vi "Trajectory Demo.vi"() -> ()   [LabVIEW 2017, in "NI_Kinematics.lvlib"]
uses:
  <vilib>/robotics/Kinematics/NI_Kinematics.lvlib
  <vilib>/robotics/Kinematics/Generate Joint Trajectory (Array).vi
  <vilib>/robotics/Kinematics/Robot/NI_Robotics_Serial Robot Arm.lvclass
panel:
  out "QDD":dbl[][](array[numeric])
  out "QD":dbl[][](array[numeric])
  out "Q":dbl[][](array[numeric])
  out "Time (ms)":u32
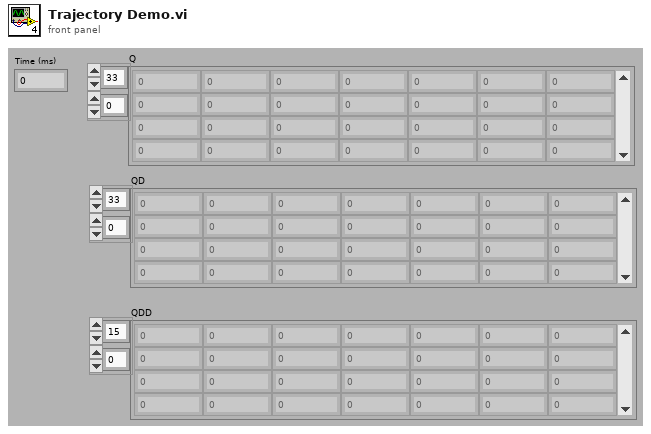
[diagram p1: front panel]
types:
  T1 = typedef "NI_Robotics_Serial Robot Arm.lvclass/Robot Pose.ctl" = cluster{"name":string, "description":string, "joint positions":dbl[]}
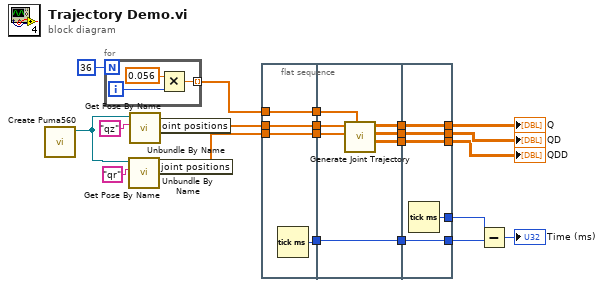
[diagram p0: block diagram]
diagram:
  n1 = call <vilib>:"Create Puma560.vi"() -> ("Puma560 Robot"=w21:refnum<class "NI_Robotics_Serial Robot Arm.lvclass">)  [unwired: 1 in, 10 out]
  n2 = for {
    N: 36 -> [_]
    tunnel: [w24] -> w12 mode=indexing
    i -> [w26]
    n3 = Multiply(x=0.056, y=w26) -> (x*y=w24:dbl)
  }
  n4 = call <vilib>:"Get Pose By Name.vi"("name"="qr" ("Name"), "serial arm in"=w21) -> ("serial arm pose"=w20:T1)  [unwired: 7 in, 2 out]
  n5 = call <vilib>:"Get Pose By Name.vi"("name"="qz" ("Name"), "serial arm in"=w21) -> ("serial arm pose"=w19:T1)  [unwired: 7 in, 2 out]
  n6 = Unbundle By Name(w19) -> ("joint positions"=w10:dbl[])
  n7 = Unbundle By Name(w20) -> ("joint positions"=w8:dbl[])
  n8 = flat-sequence {
    tunnel: [w30] -> w17
    tunnel: w12 -> [w29]
    tunnel: [w29] -> w11
    tunnel: w10 -> [w28]
    tunnel: [w28] -> w9
    tunnel: w8 -> [w27]
    tunnel: [w27] -> w7
    tunnel: w17 -> [w37]
    tunnel: [w37] -> w16
    tunnel: w11 -> [w36]
    tunnel: w9 -> [w35]
    tunnel: w7 -> [w34]
    tunnel: [w33] -> w6
    tunnel: [w32] -> w4
    tunnel: [w31] -> w3
    tunnel: [w42] -> w1
    tunnel: w16 -> [w42]
    tunnel: [w41] -> w15
    tunnel: [w40] -> w13
    tunnel: w6 -> [w40]
    tunnel: [w39] -> w5
    tunnel: w4 -> [w39]
    tunnel: w3 -> [w38]
    tunnel: [w38] -> w2
    frame #0 {
      n9 = Tick Count (ms)() -> (millisecond timer value=w30:u32)
    }
    frame #1 {
      n10 = call-poly <vilib>:"Generate Joint Trajectory.vi"("intermediate points"=w36, "end joint positions"=w34, "start joint positions"=w35) -> ("joint acceleration trajectory"=w31:dbl[][], "joint velocity trajectory"=w32:dbl[][], "joint position trajectory"=w33:dbl[][])  [unwired: 5 in, 1 out]
    }
    frame #2 {
      n11 = Tick Count (ms)() -> (millisecond timer value=w41:u32)
    }
  }
  n12 = Subtract(x=w15, y=w1) -> (x-y=→"Time (ms)":u32)
  "Q" <- w13
  "QD" <- w5
  "QDD" <- w2
